vi "AVI2-2GB split.vi"(10 "Channel":T1, 11 "Timelapse frame that couldn't be written":T2) -> (0 "error out":errorcluster)   [LabVIEW 2020]
uses:
  <vilib>/vision/Image Controls.llb/IMAQ Image.ctl
  Typedefs/Channel Selector.ctl
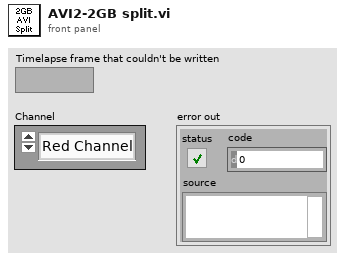
[diagram p1: front panel]
types:
  T1 = typedef "Channel Selector.ctl" = enum16{"Red Channel", "Green Channel", "Blended"}
  T2 = typedef "IMAQ Image.ctl" = refnum<image>
  T3 = typedef "Image Type" = u32
  T4 = typedef "AVI Refs cluster.ctl" = cluster{"AVI2 path":path, "AVI 2 Refnum":T5, "New Image":T2, "error out":errorcluster, "Avi 1 Refnum":T6}
  T5 = typedef "IMAQ AVI2 Refnum.ctl" = refnum<k20>
  T6 = typedef "AviRefnum.ctl" = refnum<k1>
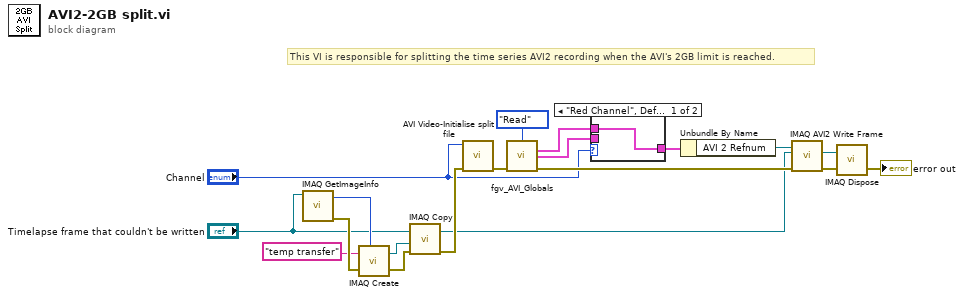
[diagram p0: block diagram]
diagram:
  # "This VI is responsible for splitting the time series AVI2 recording when the AVI's 2GB limit is reached."
  n1 = call "IMAQ GetImageInfo"("Image"="Timelapse frame that couldn't be written") -> ("error out"=w18:errorcluster, "Image Type"=w17:T3)  [unwired: 3 in, 6 out]
  n2 = call "IMAQ Create"("Image Name"="temp transfer", "Image Type"=w17, "error in (no error)"=w18) -> ("New Image"=w15:T2, "error out"=w19:errorcluster)  [unwired: 2 in]
  n3 = call "IMAQ Copy"("error in (no error)"=w19, "Image Dst"=w15, "Image Src"="Timelapse frame that couldn't be written") -> ("error out"=w13:errorcluster, "Image Dst Out"=w7:T2)  [unwired: 3 in]
  n4 = call "AVI Video-Initialise split file.vi"("error in"=w13, "Channel"="Channel") -> ("error out"=w12:errorcluster)  [unwired: 9 in]
  n5 = call "fgv_AVI_Globals.vi"("Function"=enum16{"Intialize", "Write", "Read", "Clear"}."Read", "error in (no error)"=w12) -> ("Red AVI"=w4:T4, "Green AVI"=w3:T4, "error out"=w9:errorcluster)  [unwired: 10 in, 1 out]
  n6 = case shown="\"Red Channel\", Default" "Channel" {
    tunnel: w3 -> [_ w21]
    tunnel: [w20 w21] -> w5
    tunnel: w4 -> [w20 _]
    frame "Red Channel", Default {
    }
    frame "Green Channel" {
    }
  }
  n7 = Unbundle By Name(w5) -> ("AVI 2 Refnum"=w6:T5)
  n8 = call "IMAQ AVI2 Write Frame"("error in (no error)"=w9, "Image"=w7, "AVI Refnum"=w6) -> ("error out"=w10:errorcluster, "Image Out (duplicate)"=w14:T2)  [unwired: 6 in, 1 out]
  n9 = call "IMAQ Dispose"("Image"=w14, "error in (no error)"=w10) -> ("error out"=→"error out":errorcluster)  [unwired: 4 in]
